vi "storyArcs.get.vi"(8 "error in (no error)":errorcluster, 11 "issue_class in":refnum<class "issue_class.lvclass">) -> (0 "error out":errorcluster, 1 "id":string, 2 "storyArcs":T1[](array[typedef]), 3 "issue_class out":refnum<class "issue_class.lvclass">)   [LabVIEW 2024, in "issue_class.lvclass"]
uses:
  issue_class.lvclass
  issue_class.lvclass/issue_class.ctl
  definitions/storyArc.ctl
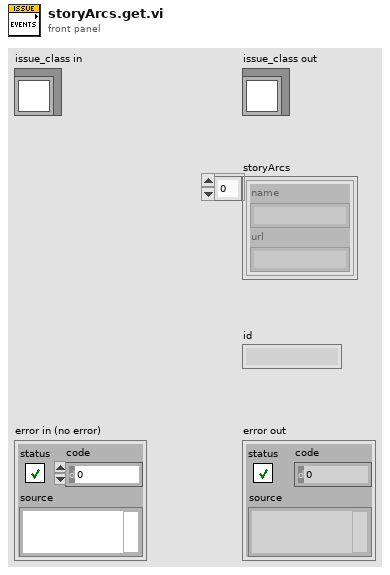
[diagram p1: front panel]
types:
  T1 = typedef "storyArc.ctl" = cluster{"name":string, "url":string}
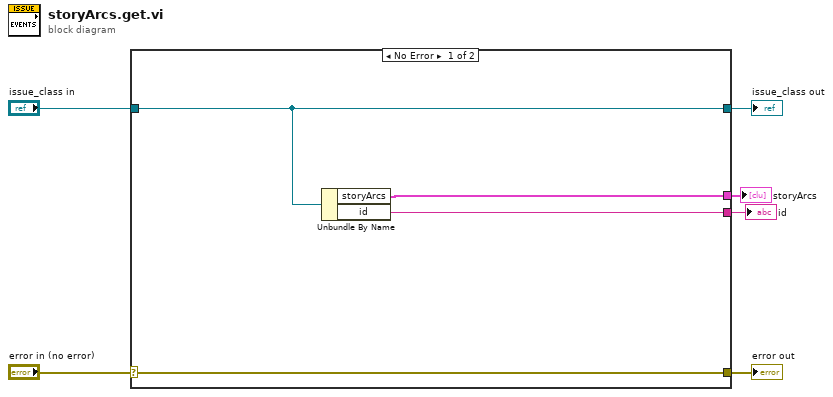
[diagram p0: block diagram]
diagram:
  n1 = case shown="No Error" "error in (no error)" {
    selector: "error in (no error)" -> [w10 w12]
    tunnel: [w10 w12] -> w5
    tunnel: [w9 w11] -> w3
    tunnel: "issue_class in" -> [w9 w11]
    tunnel: [w8 _] -> w1
    tunnel: [w7 _] -> w2
    frame No Error {
      n2 = Unbundle By Name(w9) -> ("storyArcs"=w8:T1[], "id"=w7:string)
    }
    frame Error {
    }
  }
  "error out" <- w5
  "issue_class out" <- w3
  "id" <- w2
  "storyArcs" <- w1
